vi "加+-B.vi"(1 "加B索引值":u8[](array[numeric]), 2 "加V":i8[](array[numeric])) -> (0 "加B":i8[](array[numeric]))   [LabVIEW 2013]
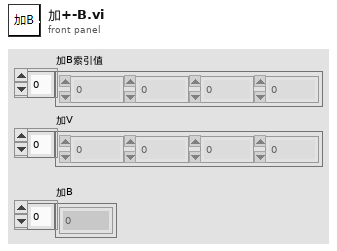
[diagram p1: front panel]
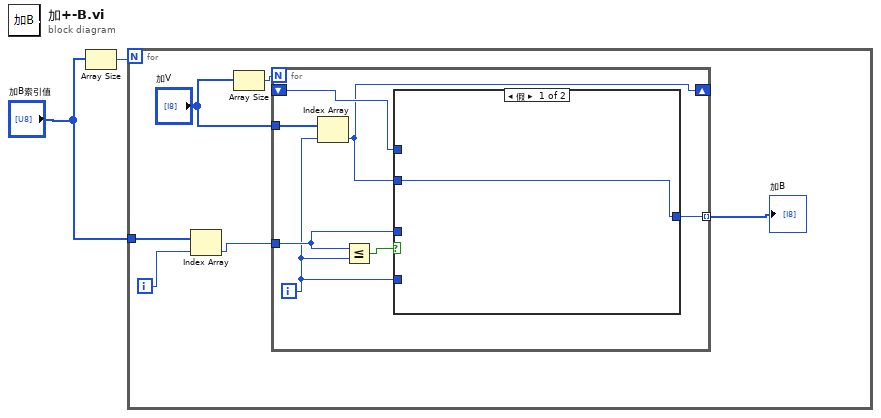
[diagram p0: block diagram]
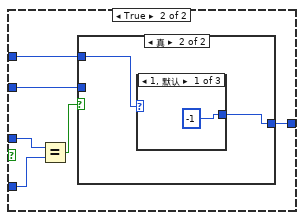
[diagram p2: hidden frame]
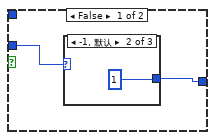
[diagram p3: hidden frame]
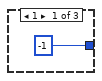
[diagram p4: hidden frame]
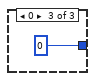
[diagram p5: hidden frame]
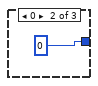
[diagram p6: hidden frame]
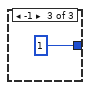
[diagram p7: hidden frame]
diagram:
  n1 = Array Size(array="加B索引值") -> (size(s)=w2:i32)
  n2 = for {
    N: w2 -> [_]
    tunnel: "加B索引值" -> [w8]
    i -> [w7]
    n3 = Index Array(array=w8, index=w7) -> (element=w4:u8)
    n4 = Array Size(array="加V") -> (size(s)=w6:i32)
    n5 = for {
      N: w6 -> [_]
      tunnel: "加V" -> [w15]
      tunnel: w4 -> [w10]
      shift-right: [w12] -> _
      shift-left: _ -> [w14]
      tunnel: [w13] -> w3 mode=indexing
      i -> [w9]
      n6 = Index Array(array=w15, index=w9) -> (element=w12:i8)
      n7 = Less Or Equal?(x=w10, y=w9) -> (x <= y?=w11:bool)
      n8 = case shown="假" w11 {
        tunnel: w14 -> [_ w22]
        tunnel: w10 -> [_ w21]
        tunnel: w9 -> [_ w20]
        tunnel: [w16 w18] -> w13
        tunnel: w12 -> [w16 w17]
        frame False {
        }
        frame True {
          n9 = Equal?(x=w21, y=w20) -> (x = y?=w19:bool)
          n10 = case shown="真" w19 {
            tunnel: w22 -> [_ w29]
            tunnel: [w23 w28] -> w18
            tunnel: w17 -> [w24 _]
            frame False {
              n11 = case shown="-1, 默认" w24 {
                tunnel: [-1 1 0] -> w23
                frame 1 {
                }
                frame -1, Default {
                }
                frame 0 {
                }
              }
            }
            frame True {
              n12 = case shown="1, 默认" w29 {
                tunnel: [-1 0 1] -> w28
                frame 1, Default {
                }
                frame 0 {
                }
                frame -1 {
                }
              }
            }
          }
        }
      }
    }
    "加B" <- w3
  }
